vi "J1939 Address Cannont Claim.vi"(0 "session out":refnum<k21>, 7 "Byte Cluster":u8[](array[numeric]), 11 "error in":errorcluster) -> (15 "error out":errorcluster)   [LabVIEW 2013, in "J1939.lvlib"]
uses:
  J1939.lvlib
  API Types/CAN Outgoing Message Cluster.ctl
  API Types/PGN Fields Cluster.ctl
  Frame Conversion/Convert J1939 ID to CAN Arb ID.vi
  <vilib>/xnet/xnet.llb/XNET Write (Frame CAN).vi
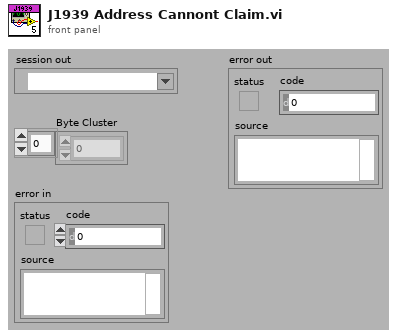
[diagram p1: front panel]
types:
  T1 = typedef "J1939.lvlib/PGN Fields Cluster.ctl" = cluster{"Reserved Bit":u8, "Data page":u8, "PDU Format":u8, "PDU Specific":u8}
  T2 = typedef "J1939.lvlib/CAN Outgoing Message Cluster.ctl" = cluster{"Identifier":u32, "Data":u8[]}
  T3 = typedef "XNET Frame CAN.ctl" = cluster{"timestamp":timestamp, "payload":u8[], "identifier":u32, "type":T4, "extended?":bool, "echo?":bool}
  T4 = typedef "XNET Frame Type CAN.ctl" = u8
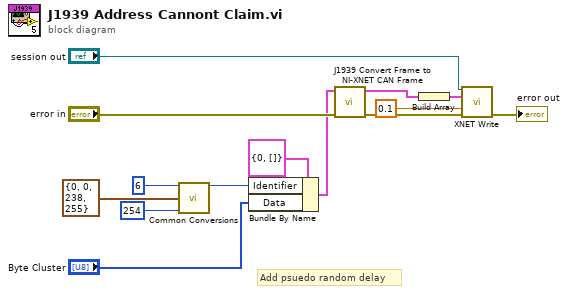
[diagram p0: block diagram]
diagram:
  # "Add psuedo random delay"
  n1 = call-poly "Common Conversions.vi"("Priority"=u8 6, "PGN Fields"=T1 {"Reserved Bit"=0, "Data page"=0, "PDU Format"=238, "PDU Specific"=255}, "Source Address"=u8 254) -> ("ID"=w3:u32)  [unwired: 2 in, 10 out]
  n2 = Bundle By Name(cluster=T2 {"Identifier"=0, "Data"=[]} ("Data to Send"), "Identifier"=w3, "Data"="Byte Cluster") -> (w7:T2)
  n3 = call "J1939 Convert Frame to NI-XNET CAN Frame.vi"("error in"="error in", "Data to Send"=w7) -> ("error out"=w9:errorcluster, "CAN frame"=w12:T3)  [unwired: 8 in]
  n4 = Build Array(w12) -> (w1:T3[])
  n5 = call-poly <vilib>:"XNET Write.vi"("session in"="session out", "data"=w1, "timeout (10)"=0.1, "error in (no error)"=w9) -> ("error out"=→"error out":errorcluster)  [unwired: 11 out]
